vi "Single stroke 2.vi"(10 "Numeric":dbl, 11 "BrickReference in":T1) -> (3 "BrickReference out":T1)   [LabVIEW 2016]
uses:
  <vilib>/NXT/Subs/LVHSConnector.ctl
  <vilib>/NXT/LegoClasses/BrickReference/BrickReference.lvclass
  <vilib>/NXT/Block Support/NXT_OutputPort.ctl
  <vilib>/NXT/NXTIO Xnodes/NXTIONodeSubVIs/NXTMoveMotors.vi
  <vilib>/NXT/Dual Mode Library/Waits/Wait_Rotation.vi
  <vilib>/NXT/NXTIO Xnodes/NXTIONodeSubVIs/LEGOStopAllMotors.vi
  <vilib>/NXT/Dual Mode Library/Waits/Wait_Num.vi
  <vilib>/NXT/NXTIO Xnodes/AddressXNode/NXTIOAddress.xnode
  <vilib>/NXT/NXTIO Xnodes/NXTIOXNode/NXTIO.xnode
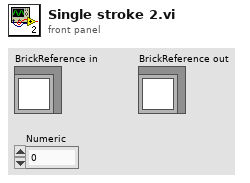
[diagram p1: front panel]
types:
  T1 = typedef "LVHSConnector.ctl" = refnum<class "BrickReference.lvclass">
  T2 = typedef "NXT_OutputPort.ctl" = u8
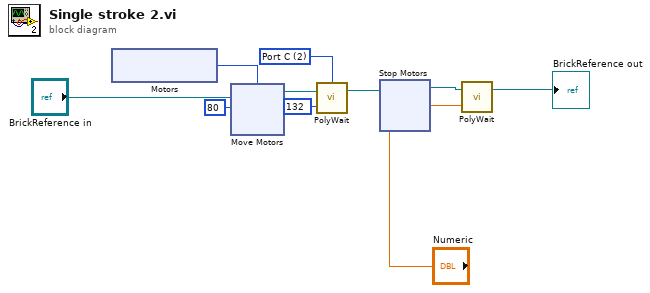
[diagram p0: block diagram]
diagram:
  w7 = T2 2 items=["Port A", "Port B", "Port C", "Port D"] ("Port (Port A)")
  n1 = xnode "Motors"() -> ("Motor"=w6:T2)
  n2 = xnode "Move Motors"("Power/Speed 1"=i8 80, "Motors"=w6, "NXT/EV3"="BrickReference in") -> ("NXT/EV3"=w4:T1)
  n3 = call-poly <vilib>:"PolyWait.vi"("Position Change (180)"=132, "NXT/EV3"=w4, "Port (Port A)"=w7) -> ("NXT/EV3"=w2:T1)  [unwired: 1 in]
  n4 = xnode "Stop Motors"("NXT/EV3"=w2) -> ("NXT/EV3"=w1:T1)  [unwired: 1 in]
  n5 = call-poly <vilib>:"PolyWait.vi"("Time (1 sec)"="Numeric", "NXT/EV3"=w1) -> ("NXT/EV3"=→"BrickReference out":T1)  [unwired: 2 in]
